vi "z bytes copy from string.vi"(8 "error in (no error)":errorcluster, 10 "str":cluster{}, 11 "this_":cluster{}) -> (0 "error out":errorcluster, 3 "this_ out":cluster{})   [LabVIEW 2021, in "zenohc.lvlib"]
doc: "void z_bytes_copy_from_string(struct z_owned_bytes_t *this_,\n const struct z_loaned_string_t *str);"
uses:
  zenohc.lvlib
  zenohc.dll
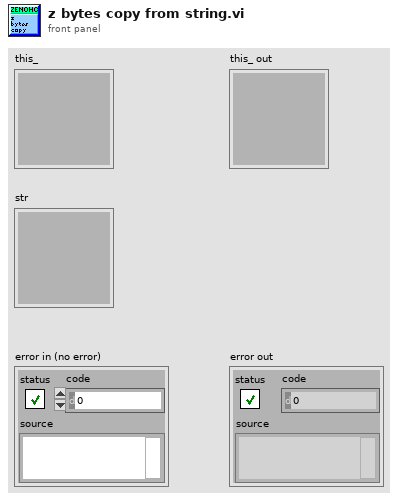
[diagram p1: front panel]
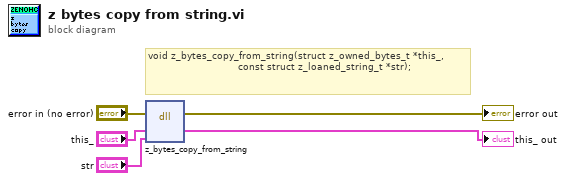
[diagram p0: block diagram]
diagram:
  # "void z_bytes_copy_from_string(struct z_owned_bytes_t *this_,\n                              const struct z_loaned_string_t *str);"
  n1 = dll-call lib="D:/dev/zenoh_labview/zenohc/zenohc.*" fn="z_bytes_copy_from_string"(error in="error in (no error)", "this_"="this_", "str"="str") -> (error out=→"error out":errorcluster, "this_"=→"this_ out":cluster{})  [unwired: 4 in, 1 out]
